vi "S_ReadWriteAttribute.vi"(8 "error in (no error)":errorcluster, 11 "reference in":refnum<class "SubTemplate_4x4x4.lvclass">) -> (0 "error out":errorcluster, 3 "reference out":refnum<class "SubTemplate_4x4x4.lvclass">)   [LabVIEW 2020]
uses:
  SubTemplate_4x4x4.lvclass
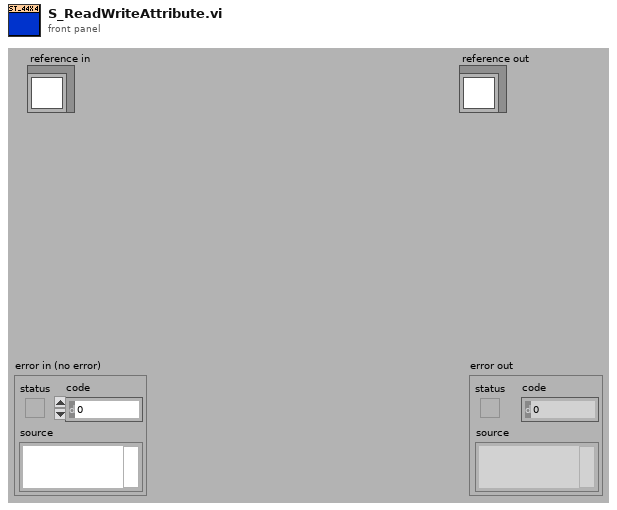
[diagram p1: front panel]
types:
  T1 = typedef "SubTemplate_4x4x4.lvclass/ObjectAttributes.ctl" = cluster{"Base class":T2}
  T2 = typedef "BaseTemplate_4x4x4.lvclass/ObjectAttributes.ctl" = cluster{"Attribute1":dbl}
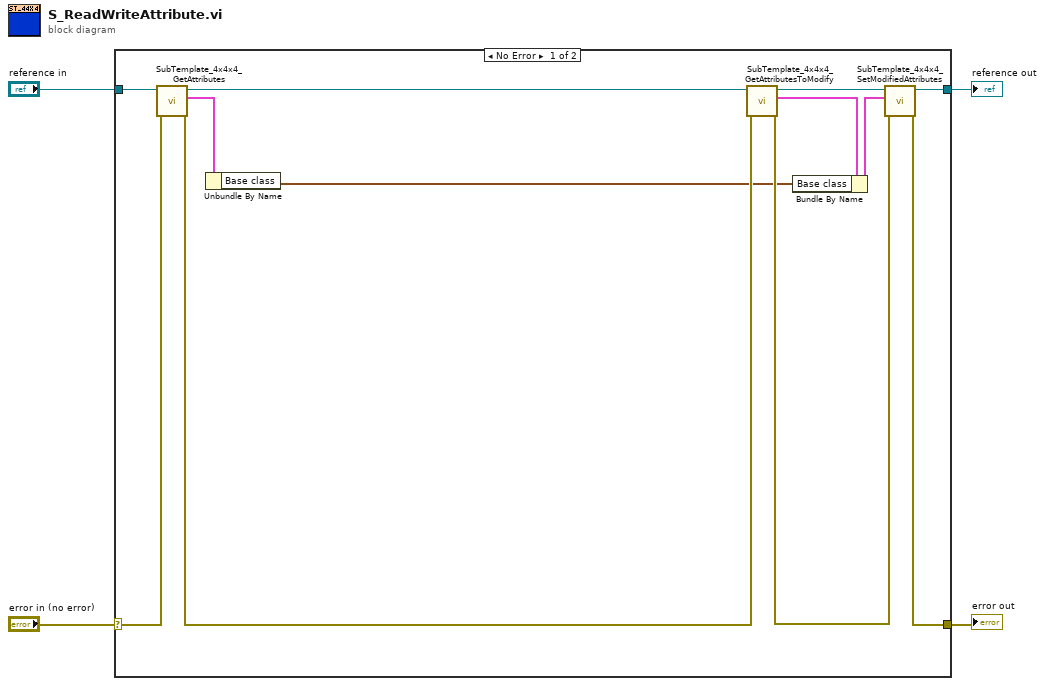
[diagram p0: block diagram]
diagram:
  n1 = case shown="No Error" "error in (no error)" {
    selector: "error in (no error)" -> [w9 w18]
    tunnel: [w13 w18] -> w3
    tunnel: [w12 w17] -> w1
    tunnel: "reference in" -> [w10 w17]
    frame No Error {
      n2 = call "SubTemplate_4x4x4_GetAttributes.vi"("error in (no error)"=w9, "reference in"=w10) -> ("error out"=w8:errorcluster, "Attributes"=w6:T1, "reference out"=w7:refnum<class "SubTemplate_4x4x4.lvclass">)  [unwired: 6 in, 1 out]
      n3 = Unbundle By Name(w6) -> ("Base class"=w5:T2)
      n4 = call "SubTemplate_4x4x4_GetAttributesToModify.vi"("error in (no error)"=w8, "reference in"=w7) -> ("error out"=w11:errorcluster, "Attributes"=w16:T1, "reference out"=w14:refnum<class "SubTemplate_4x4x4.lvclass">)  [unwired: 6 in, 1 out]
      n5 = Bundle By Name(cluster=w16, "Base class"=w5) -> (w15:T1)
      n6 = call "SubTemplate_4x4x4_SetModifiedAttributes.vi"("error in (no error)"=w11, "Attributes"=w15, "reference in"=w14) -> ("error out"=w13:errorcluster, "reference out"=w12:refnum<class "SubTemplate_4x4x4.lvclass">)  [unwired: 7 in]
    }
    frame Error {
    }
  }
  "error out" <- w3
  "reference out" <- w1
